vi "Read Heartbeat timeout.vi"(8 "error in (no error)":errorcluster, 11 "Server in":refnum<class "Server.lvclass">) -> (0 "error out":errorcluster, 2 "Heartbeat timeout":dbl caption="Heartbeat timeout [s]", 3 "Server out":refnum<class "Server.lvclass">)   [LabVIEW 2013, in "Server.lvlib" / "Server.lvclass"]
uses:
  Server.lvclass
  Server.lvclass/Server.ctl
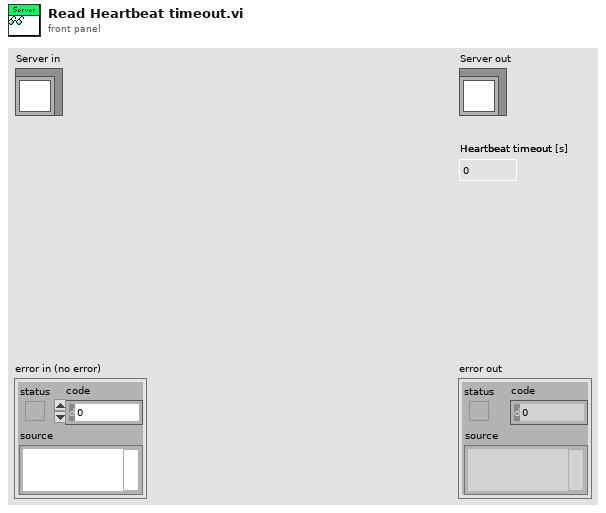
[diagram p1: front panel]
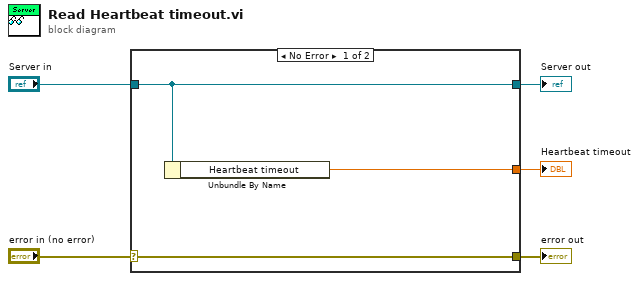
[diagram p0: block diagram]
diagram:
  n1 = case shown="No Error" "error in (no error)" {
    selector: "error in (no error)" -> [w8 w9]
    tunnel: [w8 w9] -> w4
    tunnel: [w7 w10] -> w2
    tunnel: "Server in" -> [w7 w10]
    tunnel: [w6 _] -> w1
    frame No Error {
      n2 = Unbundle By Name(w7) -> ("Heartbeat timeout"=w6:dbl)
    }
    frame Error {
    }
  }
  "error out" <- w4
  "Server out" <- w2
  "Heartbeat timeout" <- w1
